vi "Untitled 1.vi"() -> ()   [LabVIEW 2023]
uses:
  Control Timer.ctl
panel:
  in  "STOP":bool
  in  "Specijalno pranje":bool
  in  "Obicno pranje":bool
  out "error out":errorcluster
  in  "error in (no error)":errorcluster
  out "Susenje":bool
  out "Voskiranje":bool
  out "Ispiranje":bool
  out "Samponiranje":bool
  out "PranjeSasije":bool
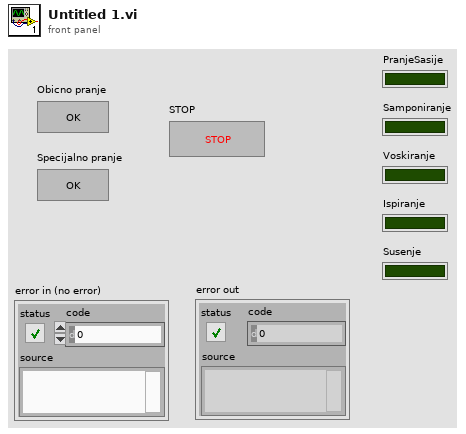
[diagram p1: front panel]
types:
  T1 = typedef "Control Timer.ctl" = enum16{"Timecheck", "Reset"}
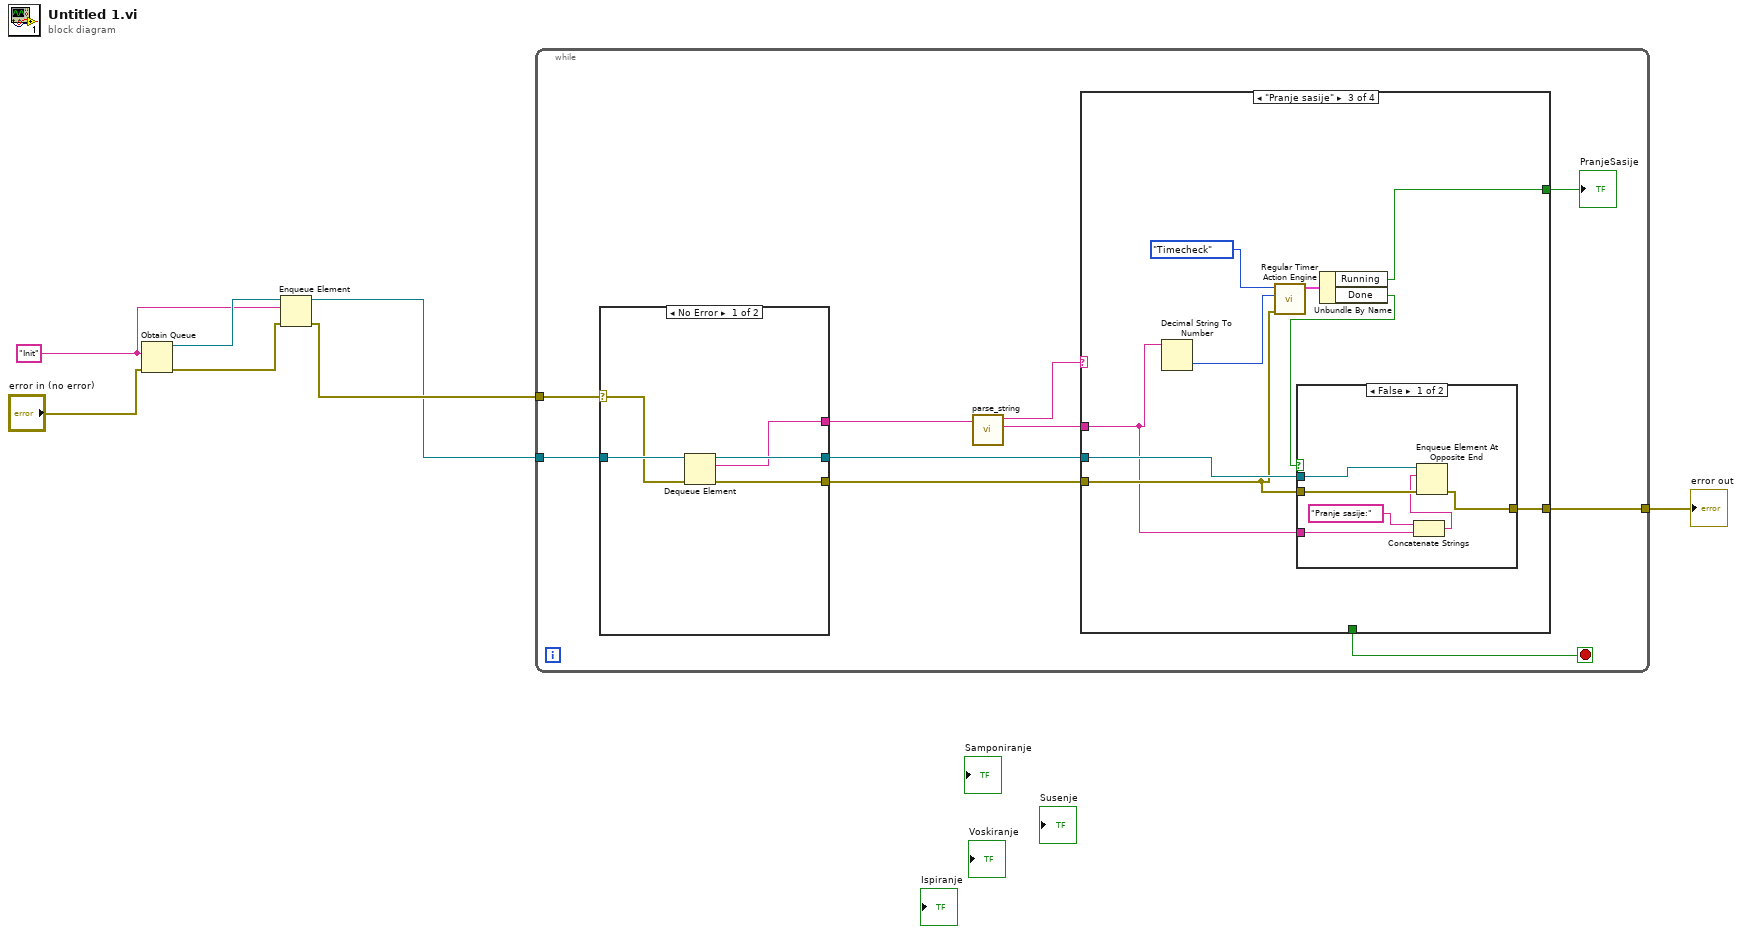
[diagram p0: block diagram]
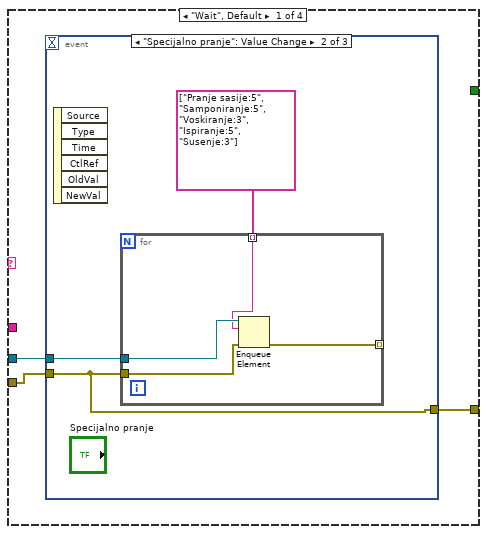
[diagram p2: hidden frame]
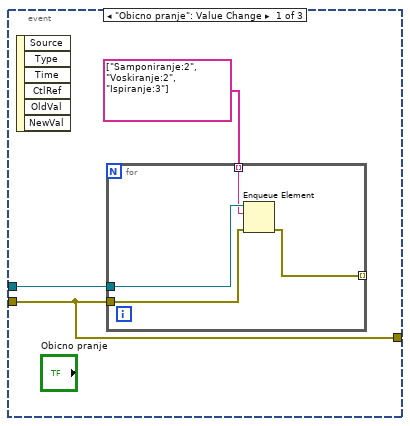
[diagram p3: hidden frame]
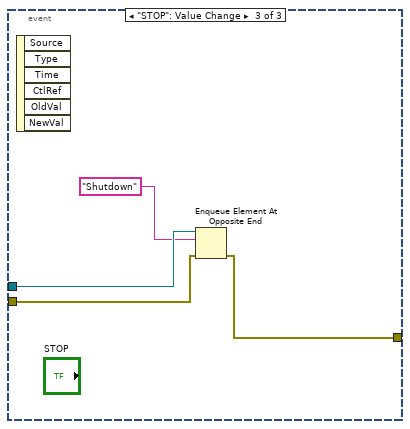
[diagram p4: hidden frame]
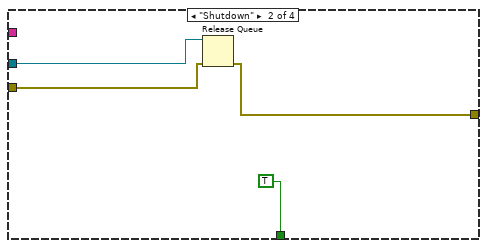
[diagram p5: hidden frame]
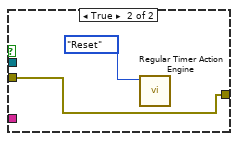
[diagram p6: hidden frame]
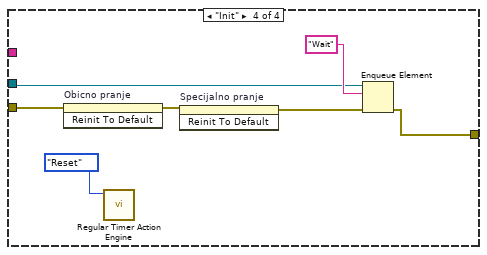
[diagram p7: hidden frame]
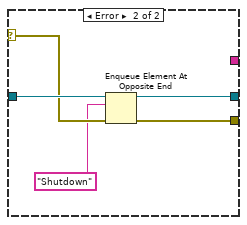
[diagram p8: hidden frame]
diagram:
  w5 = "Init"
  n1 = Obtain Queue(element data type=w5, error in (no error)="error in (no error)") -> (queue out=w6:refnum<queue>, error out=w4:errorcluster)  [unwired: 3 in, 1 out]
  n2 = Enqueue Element(queue=w6, element=w5, error in (no error)=w4) -> (queue out=w2:refnum<queue>, error out=w3:errorcluster)  [unwired: 1 in, 1 out]
  n3 = while {
    tunnel: w3 -> [w17]
    tunnel: w2 -> [w16]
    tunnel: [w10] -> w1
    stop <- w9 stop-if-true
    n4 = case shown="No Error" w17 {
      selector: w17 -> [w70 w75]
      tunnel: w16 -> [w71 w76]
      tunnel: [w68 w73] -> w11
      tunnel: [w69 w72] -> w12
      tunnel: [w67 _] -> w13
      frame No Error {
        n5 = Dequeue Element(queue=w71, error in (no error)=w70) -> (queue out=w69:refnum<queue>, element=w67:string, error out=w68:errorcluster)  [unwired: 1 in, 1 out]
      }
      frame Error {
        n6 = Enqueue Element At Opposite End(queue=w76, element="Shutdown", error in (no error)=w75) -> (queue out=w72:refnum<queue>, error out=w73:errorcluster)  [unwired: 1 in, 1 out]
      }
    }
    n7 = call "parse_string.vi"("Input"=w13) -> ("Argument"=w14:string, "Stanje"=w15:string)  [unwired: 9 in]
    n8 = case shown="\"Pranje sasije\"" w15 {
      tunnel: w14 -> [_ _ w43 _]
      tunnel: w12 -> [w20 w41 w49 w62]
      tunnel: w11 -> [w19 w42 w48 w65]
      tunnel: [w18 w40 w47 w61] -> w10
      tunnel: [_ TRUE _ _] -> w9
      tunnel: [_ _ w46 _] -> w8
      frame "Wait", Default {
        n9 = event shown="[1] \"Specijalno pranje\": Value Change" {
          selector: _ -> [_ _ _]
          dyn-events: _ -> [_ _ _]
          timeout: _ -> [_ _ _]
          tunnel: w20 -> [w23 w30 w38]
          tunnel: w19 -> [w21 w28 w37]
          tunnel: [w21 w28 w35] -> w18
          event "Obicno pranje": Value Change {
            n10 = event-data() -> ()  [unwired: 1 in, 6 out]
            n11 = for {
              tunnel: w23 -> [w27]
              tunnel: w21 -> [w26]
              tunnel: string[] ["Samponiranje:2", "Voskiranje:2", "Ispiranje:3"] -> [w25] mode=indexing
              tunnel: [w24] -> _ mode=indexing
              n12 = Enqueue Element(queue=w27, element=w25, error in (no error)=w26) -> (error out=w24:errorcluster)  [unwired: 1 in, 2 out]
            }
          }
          event "Specijalno pranje": Value Change {
            n13 = event-data() -> ()  [unwired: 1 in, 6 out]
            n14 = for {
              tunnel: w28 -> [w34]
              tunnel: w30 -> [w33]
              tunnel: string[] ["Pranje sasije:5", "Samponiranje:5", "Voskiranje:3", "Ispiranje:5", "Susenje:3"] -> [w32] mode=indexing
              tunnel: [w31] -> _ mode=indexing
              n15 = Enqueue Element(queue=w33, element=w32, error in (no error)=w34) -> (error out=w31:errorcluster)  [unwired: 1 in, 2 out]
            }
          }
          event "STOP": Value Change {
            n16 = event-data() -> ()  [unwired: 1 in, 6 out]
            n17 = Enqueue Element At Opposite End(queue=w38, element="Shutdown", error in (no error)=w37) -> (error out=w35:errorcluster)  [unwired: 1 in, 2 out]
          }
        }
      }
      frame "Shutdown" {
        n18 = Release Queue(queue=w41, error in (no error)=w42) -> (error out=w40:errorcluster)  [unwired: 1 in, 2 out]
      }
      frame "Pranje sasije" {
        n19 = Decimal String To Number(string=w43) -> (number=w45:i32)  [unwired: 2 in, 1 out]
        n20 = call "Regular Timer Action Engine.vi"("Enum"=Control_Timer."Timecheck", "Time Target"=w45, "error in"=w48) -> ("Status"=w50:cluster{"Running":bool, "Done":bool})  [unwired: 6 in, 1 out]
        n21 = Unbundle By Name(w50) -> ("Running"=w46:bool, "Done"=w44:bool)
        n22 = case shown="False" w44 {
          tunnel: w49 -> [w57 _]
          tunnel: w48 -> [w56 w58]
          tunnel: [w55 w58] -> w47
          tunnel: w43 -> [w54 _]
          frame False {
            n23 = Concatenate Strings("Pranje sasije:" ("element"), w54) -> (w52:string)
            n24 = Enqueue Element At Opposite End(queue=w57, element=w52, error in (no error)=w56) -> (error out=w55:errorcluster)  [unwired: 1 in, 2 out]
          }
          frame True {
            n25 = call "Regular Timer Action Engine.vi"("Enum"=Control_Timer."Reset") -> ()  [unwired: 8 in, 2 out]
          }
        }
      }
      frame "Init" {
        n26 = invoke on="Obicno pranje" class="Bool" method="Reinit To Default"(error in=w65) -> (error out=w64:errorcluster)  [unwired: 2 in, 2 out]
        n27 = call "Regular Timer Action Engine.vi"("Enum"=Control_Timer."Reset") -> ()  [unwired: 8 in, 2 out]
        n28 = invoke on="Specijalno pranje" class="Bool" method="Reinit To Default"(error in=w64) -> (error out=w63:errorcluster)  [unwired: 2 in, 2 out]
        n29 = Enqueue Element(queue=w62, element="Wait", error in (no error)=w63) -> (error out=w61:errorcluster)  [unwired: 1 in, 2 out]
      }
    }
    "PranjeSasije" <- w8
  }
  "error out" <- w1
